vi "CLD 10 Step Sequencer with CSV Front Panel.vi"() -> ()   [LabVIEW 2018]
doc: "CLD 10 Exercise"
uses:
  CLD 10 CSV file read eum.ctl
  CLD 10 CSV file enum.ctl
panel:
  out "Step 3":bool
  out "Current Step time":dbl
  out "Step 2":bool
  out "Step 1":bool
  out "Time Has Elapsed":bool
  out "Elapsed Time (s)":string
  in  "Auto Reset":bool=TRUE
  in  "Reset Button":bool
  in  "Stop VI":bool
  out "error out":errorcluster
  in  "error in (no error)":errorcluster
  in  "Time Target (s)":dbl
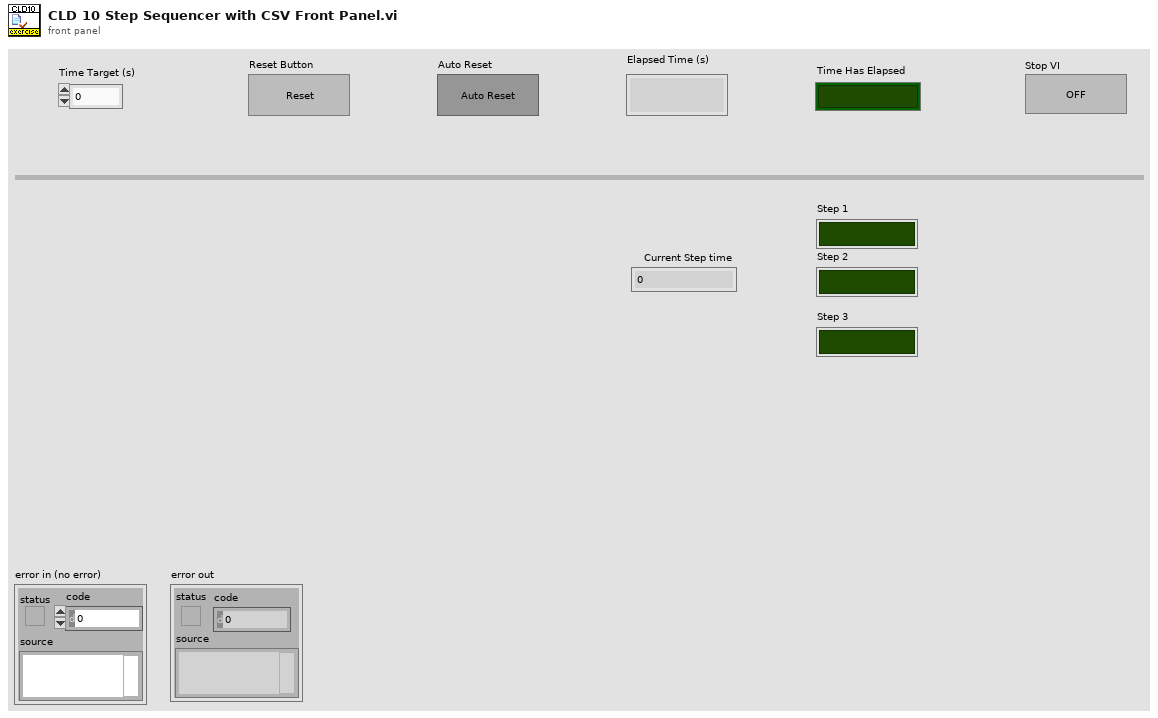
[diagram p1: front panel]
types:
  T1 = typedef "CLD 10 CSV file read eum.ctl" = enum16{"Read CSV File", "Run Step One", "Run Step Two", "Run Step Three"}
  T2 = typedef "CLD 10 CSV file enum.ctl" = enum16{"Read CSV", "Write CSV"}
  T3 = typedef "CLD 10 CSV file data structure.ctl" = cluster{"Step Time Target":i32, "Step 1":bool, "Step 2":bool, "Step 3":bool}
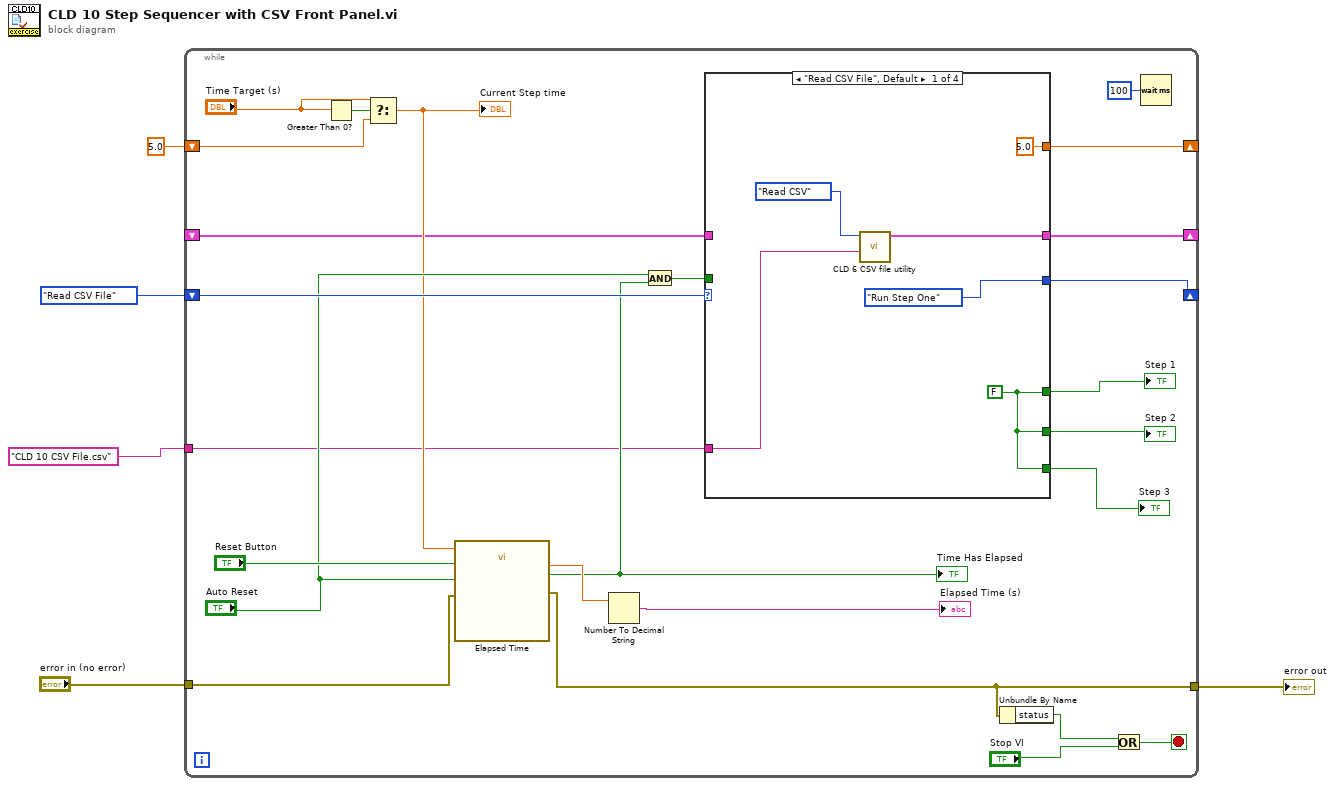
[diagram p0: block diagram]
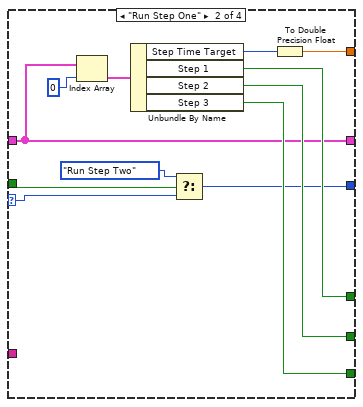
[diagram p2: hidden frame]
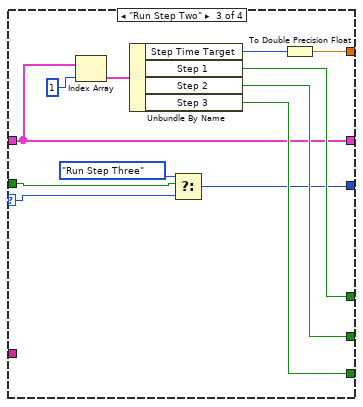
[diagram p3: hidden frame]
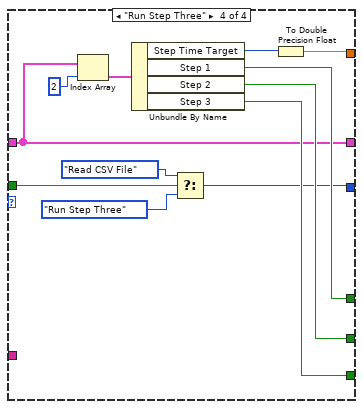
[diagram p4: hidden frame]
diagram:
  n1 = while {
    shift-right: [w8] -> _
    shift-left: CLD_10_CSV_file_read_eum."Read CSV File" ("CLD 10 Timer Enum") -> [w30]
    shift-right: [w27] -> _
    shift-left: 5.0 ("f") -> [w28]
    tunnel: "error in (no error)" -> [w26]
    tunnel: [w25] -> w3
    tunnel: "CLD 10 CSV File.csv" ("name or relative path") -> [w10]
    shift-right: [w9] -> _
    shift-left: _ -> [w7]
    stop <- w23 stop-if-true
    n2 = Greater Than 0?(x="Time Target (s)") -> (x > 0?=w29:bool)
    n3 = Select(t="Time Target (s)", s=w29, f=w28) -> (s? t:f=w11:dbl)
    "Current Step time" <- w11
    n4 = call "Elapsed Time"("Time Target (s)"=w11, "Reset"="Reset Button", "Auto Reset"="Auto Reset", "error in (no error)"=w26) -> ("Elapsed Time (s)"=w20:dbl, "Time has Elapsed"=w17:bool, "error out"=w25:errorcluster)  [unwired: 8 in, 5 out]
    "Time Has Elapsed" <- w17
    n5 = Number To Decimal String(number=w20) -> (decimal integer string=→"Elapsed Time (s)":string)  [unwired: 1 in]
    n6 = And(x="Auto Reset", y=w17) -> (x .and. y?=w21:bool)
    n7 = case shown="\"Read CSV File\", Default" w30 {
      selector: w30 -> [_ w41 w52 _]
      tunnel: w21 -> [_ w42 w53 w64]
      tunnel: [5.0 w37 w49 w62] -> w27
      tunnel: [w32 w46 w58 w70] -> w18
      tunnel: [w32 w45 w57 w69] -> w19
      tunnel: [w32 w44 w56 w68] -> w6
      tunnel: w10 -> [w35 _ _ _]
      tunnel: [w34 w43 w54 w65] -> w9
      tunnel: [CLD_10_CSV_file_read_eum."Run Step One" ("CLD 10 Timer Enum") w39 w51 w67] -> w8
      tunnel: w7 -> [_ w43 w54 w65]
      frame "Read CSV File", Default {
        w32 = FALSE
        n8 = call "CLD 6 CSV file utility.vi"("name or relative path"=w35, "CSV File Enum"=CLD_10_CSV_file_enum."Read CSV") -> ("[Data Out]"=w34:T3[])  [unwired: 8 in, 1 out]
      }
      frame "Run Step One" {
        n9 = Index Array(array=w43, index=0) -> (element=w47:T3)
        n10 = Unbundle By Name(w47) -> ("Step Time Target"=w38:i32, "Step 1"=w46:bool, "Step 2"=w45:bool, "Step 3"=w44:bool)
        n11 = Select(t=CLD_10_CSV_file_read_eum."Run Step Two" ("CLD 10 Timer Enum"), s=w42, f=w41) -> (s? t:f=w39:T1)
        n12 = To Double Precision Float(number=w38) -> (double precision float=w37:dbl)
      }
      frame "Run Step Two" {
        n13 = Index Array(array=w54, index=1) -> (element=w55:T3)
        n14 = Unbundle By Name(w55) -> ("Step Time Target"=w50:i32, "Step 1"=w58:bool, "Step 2"=w57:bool, "Step 3"=w56:bool)
        n15 = Select(t=CLD_10_CSV_file_read_eum."Run Step Three" ("CLD 10 Timer Enum"), s=w53, f=w52) -> (s? t:f=w51:T1)
        n16 = To Double Precision Float(number=w50) -> (double precision float=w49:dbl)
      }
      frame "Run Step Three" {
        n17 = Index Array(array=w65, index=2) -> (element=w66:T3)
        n18 = Unbundle By Name(w66) -> ("Step Time Target"=w63:i32, "Step 1"=w70:bool, "Step 2"=w69:bool, "Step 3"=w68:bool)
        n19 = Select(t=CLD_10_CSV_file_read_eum."Read CSV File" ("CLD 10 Timer Enum"), s=w64, f=CLD_10_CSV_file_read_eum."Run Step Three" ("CLD 10 Timer Enum")) -> (s? t:f=w67:T1)
        n20 = To Double Precision Float(number=w63) -> (double precision float=w62:dbl)
      }
    }
    "Step 1" <- w18
    "Step 2" <- w19
    "Step 3" <- w6
    n21 = Unbundle By Name(w25) -> ("status"=w24:bool)
    n22 = Or(x=w24, y="Stop VI") -> (x .or. y?=w23:bool)
    n23 = Wait (ms)(milliseconds to wait=u32 100) -> ()  [unwired: 1 out]
  }
  "error out" <- w3
